vi "Get_Ch_Time_Trace.vi"(0 "Desired Ch Names":string[](array[string]), 1 "History Length (mins)":dbl) -> (2 "Centre Times":dbl[](array[numeric]) format="%.2f", 3 "Averaging Period":dbl[](array[numeric]) format="%.2f", 4 "Output array":dbl[][](array[numeric]) format="%.2f")   [LabVIEW 2010]
uses:
  Sub VIs/ADAM Controls/Search_mode.ctl
  Sub VIs/ADAM Controls/Channel_names.ctl
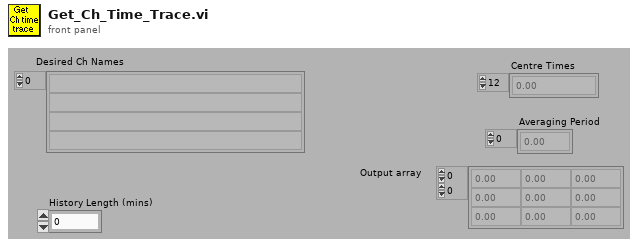
[diagram p1: front panel]
types:
  T1 = typedef "Search_mode.ctl" = enum16{"Between times", "All Times"}
  T2 = typedef "Channel_names.ctl" = enum16{"Active Only", "Active + Off", "All Channels"}
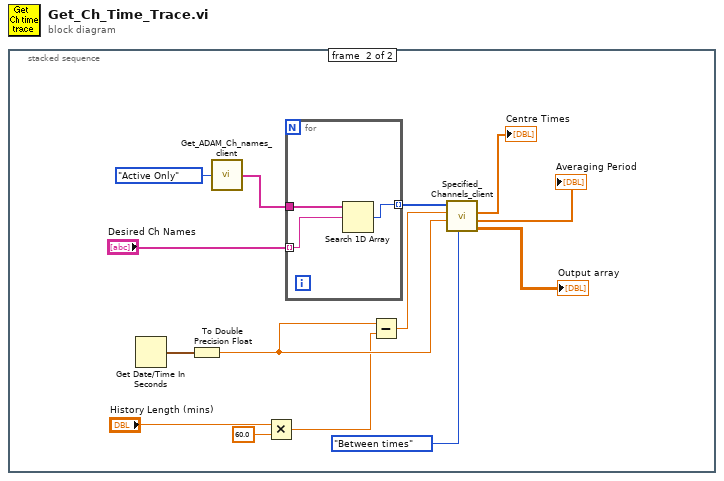
[diagram p0: block diagram]
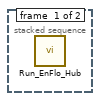
[diagram p2: hidden frame]
diagram:
  n1 = stacked-sequence {
    frame #0 {
      n2 = call "Run_EnFlo_Hub.vi"() -> ()  [unwired: 8 out]
    }
    frame #1 {
      n3 = Get Date/Time In Seconds() -> (seconds since 1Jan1904=w10:timestamp)
      n4 = To Double Precision Float(number=w10) -> (double precision float=w7:dbl)
      n5 = call "Get_ADAM_Ch_names_client.vi"("Channel names set"=Channel_names."Active Only") -> ("Ch names"=w14:string[])
      n6 = Multiply(x="History Length (mins)", y=60.0) -> (x*y=w6:dbl)
      n7 = for {
        tunnel: w14 -> [w17]
        tunnel: "Desired Ch Names" -> [w16] mode=indexing
        tunnel: [w15] -> w11 mode=indexing
        n8 = Search 1D Array(1D array=w17, element=w16) -> (index of element=w15:i32)  [unwired: 1 out]
      }
      n9 = Subtract(x=w7, y=w6) -> (x-y=w5:dbl)
      n10 = call "Specified_Channels_client.vi"("Mode"=Search_mode."Between times", "End time"=w7, "Start time"=w5, "ADAM Index array"=w11) -> ("Output array"=→"Output array":dbl[][], "Averaging Period"=→"Averaging Period":dbl[], "Centre Times"=→"Centre Times":dbl[])  [unwired: 5 out]
    }
  }
